vi "ReadData.vi"(8 "error in":errorcluster, 11 "Module Config Selector":i16) -> (0 "error out":errorcluster, 3 "Data Array":sgl[](array[numeric]) format="%.2f")   [LabVIEW 2017, in "BOP_VibAPI_4.lvlib"]
uses:
  <vilib>/addons/InsightCM/Devices/Shared/Cms/Fpga/Acquisition/source/subVIs/VibAPI_4/BOP_VibAPI_4.lvlib
  <vilib>/rvi/eio/common/nirviEmuTemplateMethod_errors.vi
  <vilib>/eio/EIONode/EIONode.xnode
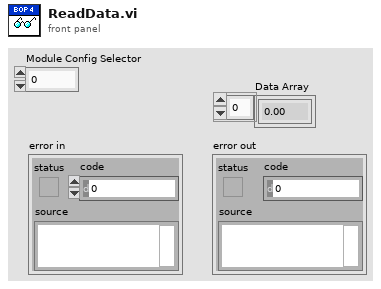
[diagram p1: front panel]
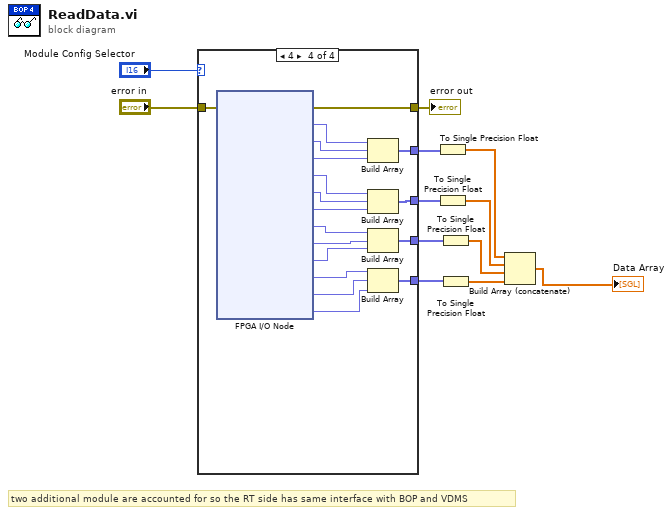
[diagram p0: block diagram]
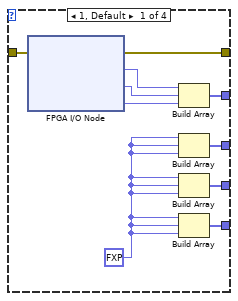
[diagram p2: hidden frame]
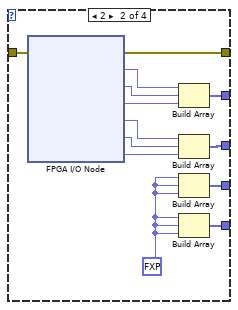
[diagram p3: hidden frame]
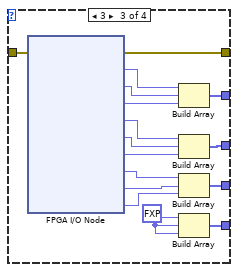
[diagram p4: hidden frame]
diagram:
  # "two additional module are accounted for so the RT side has same interface with BOP and VDMS"
  n1 = case shown="4" "Module Config Selector" {
    tunnel: "error in" -> [w19 w32 w48 w66]
    tunnel: [w18 w31 w47 w65] -> w11
    tunnel: [w17 w30 w46 w64] -> w8
    tunnel: [w16 w29 w45 w63] -> w6
    tunnel: [w15 w28 w44 w62] -> w4
    tunnel: [w14 w24 w37 w52] -> w2
    frame 1, Default {
      w13 = fxp<+/-,24,7> 0.0 ("Mod1/AI2")
      n2 = xnode "FPGA I/O Node"("error in"=w19) -> ("error out"=w18:errorcluster, "Mod1/AI0"=w20:fxp<+/-,24,7>, "Mod1/AI1"=w22:fxp<+/-,24,7>, "Mod1/AI2"=w21:fxp<+/-,24,7>)  [unwired: 3 in, 3 out]
      n3 = Build Array(w20, w22, w21) -> (w17:fxp<+/-,24,7>[])
      n4 = Build Array(w13, w13, w13) -> (w16:fxp<+/-,24,7>[])
      n5 = Build Array(w13, w13, w13) -> (w15:fxp<+/-,24,7>[])
      n6 = Build Array(w13, w13, w13) -> (w14:fxp<+/-,24,7>[])
    }
    frame 2 {
      w23 = fxp<+/-,24,7> 0.0 ("Mod3/AI0")
      n7 = xnode "FPGA I/O Node"("error in"=w32) -> ("error out"=w31:errorcluster, "Mod1/AI0"=w33:fxp<+/-,24,7>, "Mod1/AI1"=w35:fxp<+/-,24,7>, "Mod1/AI2"=w34:fxp<+/-,24,7>, "Mod2/AI0"=w27:fxp<+/-,24,7>, "Mod2/AI1"=w26:fxp<+/-,24,7>, "Mod2/AI2"=w25:fxp<+/-,24,7>)  [unwired: 6 in, 6 out]
      n8 = Build Array(w33, w35, w34) -> (w30:fxp<+/-,24,7>[])
      n9 = Build Array(w27, w26, w25) -> (w29:fxp<+/-,24,7>[])
      n10 = Build Array(w23, w23, w23) -> (w28:fxp<+/-,24,7>[])
      n11 = Build Array(w23, w23, w23) -> (w24:fxp<+/-,24,7>[])
    }
    frame 3 {
      w36 = fxp<+/-,24,7> 0.0 ("Mod3/AI2")
      n12 = xnode "FPGA I/O Node"("error in"=w48) -> ("error out"=w47:errorcluster, "Mod1/AI0"=w49:fxp<+/-,24,7>, "Mod1/AI1"=w51:fxp<+/-,24,7>, "Mod1/AI2"=w50:fxp<+/-,24,7>, "Mod2/AI0"=w43:fxp<+/-,24,7>, "Mod2/AI1"=w42:fxp<+/-,24,7>, "Mod2/AI2"=w41:fxp<+/-,24,7>, "Mod3/AI0"=w40:fxp<+/-,24,7>, "Mod3/AI1"=w39:fxp<+/-,24,7>, "Mod3/AI2"=w38:fxp<+/-,24,7>)  [unwired: 9 in, 9 out]
      n13 = Build Array(w49, w51, w50) -> (w46:fxp<+/-,24,7>[])
      n14 = Build Array(w43, w42, w41) -> (w45:fxp<+/-,24,7>[])
      n15 = Build Array(w40, w39, w38) -> (w44:fxp<+/-,24,7>[])
      n16 = Build Array(w36, w36, w36) -> (w37:fxp<+/-,24,7>[])
    }
    frame 4 {
      n17 = xnode "FPGA I/O Node"("error in"=w66) -> ("error out"=w65:errorcluster, "Mod1/AI0"=w67:fxp<+/-,24,7>, "Mod1/AI1"=w69:fxp<+/-,24,7>, "Mod1/AI2"=w68:fxp<+/-,24,7>, "Mod2/AI0"=w61:fxp<+/-,24,7>, "Mod2/AI1"=w60:fxp<+/-,24,7>, "Mod2/AI2"=w59:fxp<+/-,24,7>, "Mod3/AI0"=w58:fxp<+/-,24,7>, "Mod3/AI1"=w57:fxp<+/-,24,7>, "Mod3/AI2"=w56:fxp<+/-,24,7>, "Mod4/AI0"=w55:fxp<+/-,24,7>, "Mod4/AI1"=w54:fxp<+/-,24,7>, "Mod4/AI2"=w53:fxp<+/-,24,7>)  [unwired: 12 in, 12 out]
      n18 = Build Array(w67, w69, w68) -> (w64:fxp<+/-,24,7>[])
      n19 = Build Array(w61, w60, w59) -> (w63:fxp<+/-,24,7>[])
      n20 = Build Array(w58, w57, w56) -> (w62:fxp<+/-,24,7>[])
      n21 = Build Array(w55, w54, w53) -> (w52:fxp<+/-,24,7>[])
    }
  }
  "error out" <- w11
  n22 = To Single Precision Float(number=w8) -> (single precision float=w7:sgl[])
  n23 = To Single Precision Float(number=w6) -> (single precision float=w5:sgl[])
  n24 = To Single Precision Float(number=w4) -> (single precision float=w3:sgl[])
  n25 = To Single Precision Float(number=w2) -> (single precision float=w1:sgl[])
  n26 = Build Array (concatenate)(w7, w5, w3, w1) -> (→"Data Array":sgl[])
